vi "PIDExitWhenStable.vi"(0 "NewValue":dbl, 1 "Iterations":i32=1000, 2 "Threshold":dbl=0.1, 4 "DelayIterations":i32=200, 5 "CurrentIteration":i32) -> (7 "ShouldExit?":bool)   [LabVIEW 2016]
uses:
  <vilib>/ptbypt/NI_PtbyPt.lvlib
panel:
  in  "Timeout":dbl=inf
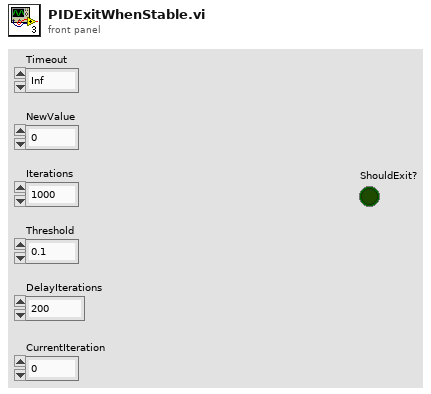
[diagram p1: front panel]
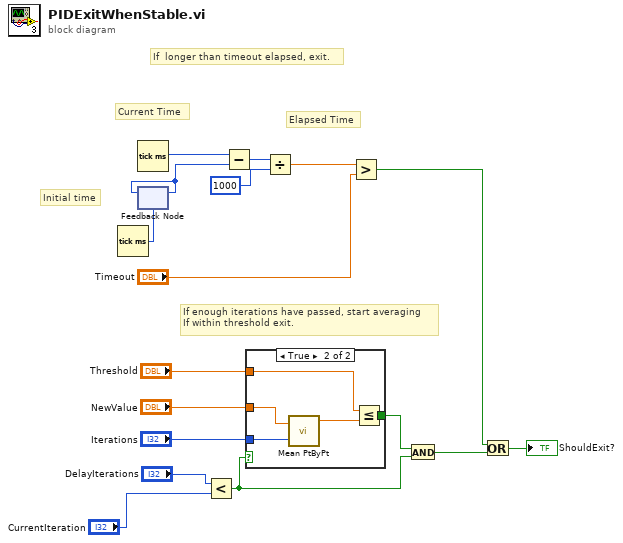
[diagram p0: block diagram]
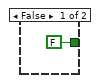
[diagram p2: hidden frame]
diagram:
  # "If  longer than timeout elapsed, exit."
  # "If enough iterations have passed, start averaging\nIf within threshold exit."
  # "Elapsed Time"
  # "Current Time"
  # "Initial time"
  n1 = Tick Count (ms)() -> (millisecond timer value=w11:u32)
  n2 = Tick Count (ms)() -> (millisecond timer value=w10:u32)
  n3 = feedback #1(w11) -> (w9:u32)
  n4 = feedback-in #1(w9) -> ()
  n5 = Less?(x="DelayIterations", y="CurrentIteration") -> (x < y?=w12:bool)
  n6 = Subtract(x=w10, y=w9) -> (x-y=w7:u32)
  n7 = case shown="True" w12 {
    tunnel: "Iterations" -> [_ w23]
    tunnel: "NewValue" -> [_ w22]
    tunnel: "Threshold" -> [_ w21]
    tunnel: [FALSE w19] -> w13
    frame False {
    }
    frame True {
      n8 = call <vilib>:"Mean PtByPt.vi"("x"=w22, "sample length"=w23) -> ("mean"=w20:dbl)  [unwired: 2 in, 1 out]
      n9 = Less Or Equal?(x=w21, y=w20) -> (x <= y?=w19:bool)
    }
  }
  n10 = Divide(x=w7, y=u32 1000) -> (x/y=w5:dbl)
  n11 = Greater?(x=w5, y="Timeout") -> (0:w2:bool)
  n12 = And(x=w13, y=w12) -> (x .and. y?=w3:bool)
  n13 = Or(x=w2, y=w3) -> (x .or. y?=→"ShouldExit?":bool)
